vi "Calculate Pulse Width.vi"(9 "Channel":i32, 11 "Samples":dbl[](array[numeric])) -> (3 "Pulse Width":dbl)   [LabVIEW 2010]
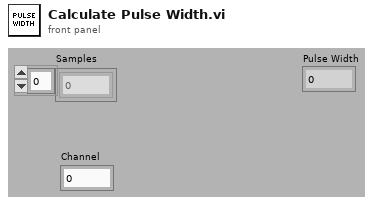
[diagram p1: front panel]
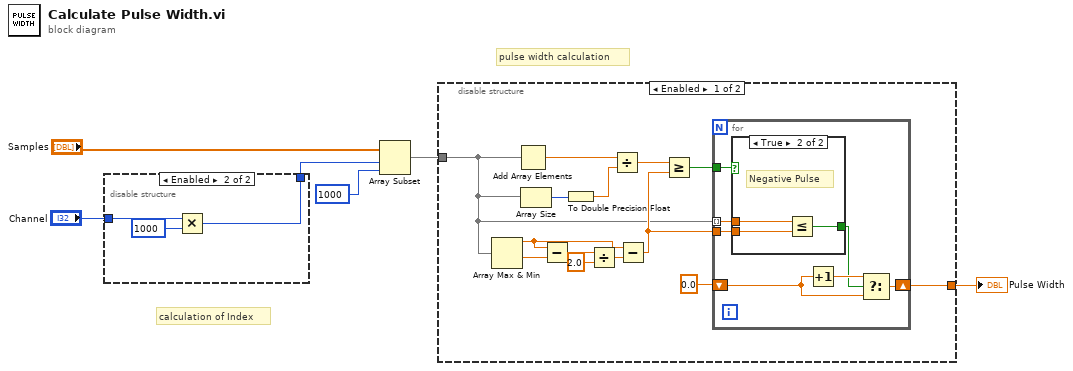
[diagram p0: block diagram]
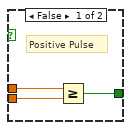
[diagram p2: hidden frame]
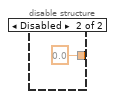
[diagram p3: hidden frame]
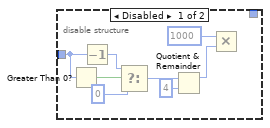
[diagram p4: hidden frame]
diagram:
  # "pulse width calculation"
  # "calculation of Index"
  n1 = disable-structure shown="Enabled" {
    disable-tunnel: "Channel" -> [w11 w17]
    disable-tunnel: [_ w15] -> w4
    frame Disabled {
      n2 = Greater Than 0?(x=w11) -> (x > 0?=w10:bool)
      n3 = Decrement(x=w11) -> (x-1=w9:i32)
      n4 = Select(t=w9, s=w10, f=u32 0) -> (s? t:f=w8:u32)
      n5 = Quotient & Remainder(x=w8, y=u32 4) -> (x-y*floor(x/y)=w13:u32)  [unwired: 1 out]
      n6 = Multiply(x=u32 1000, y=w13) -> ()  [unwired: 1 out]
    }
    frame Enabled {
      n7 = Multiply(x=w17, y=1000) -> (x*y=w15:i32)
    }
  }
  n8 = Array Subset(array="Samples", index=w4, length=1000 ("x")) -> (w2:dbl[])
  n9 = disable-structure shown="Enabled" {
    disable-tunnel: w2 -> [w20 _]
    disable-tunnel: [w19 0.0 ("Pulse Width")] -> w1
    frame Enabled {
      n10 = Array Max & Min(array=w20) -> (max value=w27:dbl, min value=w31:dbl)  [unwired: 2 out]
      n11 = Add Array Elements(numeric array=w20) -> (sum=w26:dbl)
      n12 = Array Size(array=w20) -> (size(s)=w21:i32)
      n13 = Subtract(x=w27, y=w31) -> (x-y=w28:dbl)
      n14 = To Double Precision Float(number=w21) -> (double precision float=w18:dbl)
      n15 = Divide(x=w28, y=2.0) -> (x/y=w29:dbl)
      n16 = Divide(x=w26, y=w18) -> (x/y=w24:dbl)
      n17 = Subtract(x=w27, y=w29) -> (x-y=w22:dbl)
      n18 = Greater Or Equal?(x=w24, y=w22) -> (x >= y?=w25:bool)
      n19 = for {
        tunnel: w25 -> [w38]
        tunnel: w20 -> [w37] mode=indexing
        tunnel: w22 -> [w36]
        shift-right: [w35] -> w19
        shift-left: 0.0 ("index") -> [w33]
        n20 = case shown="True" w38 {
          tunnel: w37 -> [w40 w44]
          tunnel: w36 -> [w39 w43]
          tunnel: [w41 w42] -> w32
          frame False {
            # "Positive Pulse"
            n21 = Greater Or Equal?(x=w40, y=w39) -> (x >= y?=w41:bool)
          }
          frame True {
            # "Negative Pulse"
            n22 = Less Or Equal?(x=w44, y=w43) -> (x <= y?=w42:bool)
          }
        }
        n23 = Increment(x=w33) -> (x+1=w34:dbl)
        n24 = Select(t=w34, s=w32, f=w33) -> (s? t:f=w35:dbl)
      }
    }
    frame Disabled {
    }
  }
  "Pulse Width" <- w1
